vi "G4SubTemplate_Simple_4x4x4_ReadWriteAttribute.vi"(8 "Error In":errorcluster, 11 "reference in":refnum<class "G4SubTemplate_Simple_4x4x4.lvclass">) -> (0 "Error Out":errorcluster, 3 "reference in":refnum<class "G4SubTemplate_Simple_4x4x4.lvclass">)   [LabVIEW 2020]
uses:
  <resource>/Framework/Providers/Open_GDS/ClassProviders/Provider_EndevoGOOP400/Templates/G4SubTemplate_Simple_4x4x4/G4SubTemplate_Simple_4x4x4.lvclass
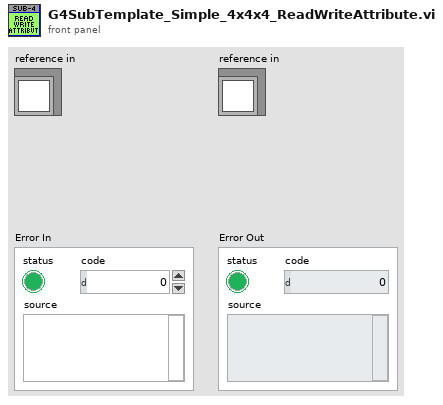
[diagram p1: front panel]
types:
  T1 = typedef "G4SubTemplate_Simple_4x4x4.lvclass/ObjectAttribute.ctl" = cluster{"Attribute1":dbl}
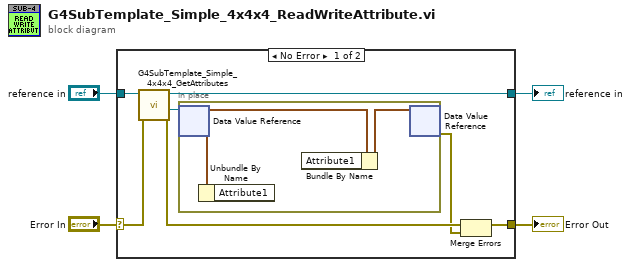
[diagram p0: block diagram]
diagram:
  n1 = case shown="No Error" "Error In" {
    selector: "Error In" -> [w10 w15]
    tunnel: [w9 w15] -> w3
    tunnel: [w8 w14] -> w1
    tunnel: "reference in" -> [w11 w14]
    frame No Error {
      n2 = call <resource>:"G4SubTemplate_Simple_4x4x4_GetAttributes.vi"("error in (no error)"=w10, "reference in"=w11) -> ("error out"=w6:errorcluster, "DataRef"=w7:refnum<data-value>, "reference out"=w8:refnum<class "G4SubTemplate_Simple_4x4x4.lvclass">)  [unwired: 6 in, 1 out]
      n3 = in-place {
        n4 = in-place-dvr #1(w7) -> (w12:T1)  [unwired: 1 out]
        n5 = Unbundle By Name(w12) -> ()  [unwired: 1 out]
        n6 = Bundle By Name(cluster=w12) -> (w13:T1)  [unwired: 1 in]
        n7 = in-place-dvr #1(w13) -> (w5:errorcluster)  [unwired: 1 out]
      }
      n8 = Merge Errors(w6, w5) -> (w9:errorcluster)
    }
    frame Error {
    }
  }
  "Error Out" <- w3
  "reference in" <- w1
